vi "FisherPaykel Check GEA Inverter Selection.vi"(8 "Error In":errorcluster, 10 "Inverter ID":string(combo), 11 "Machine ID":string(combo)) -> (0 "Error Out":errorcluster, 3 "Throw Error?":bool)   [LabVIEW 2016]
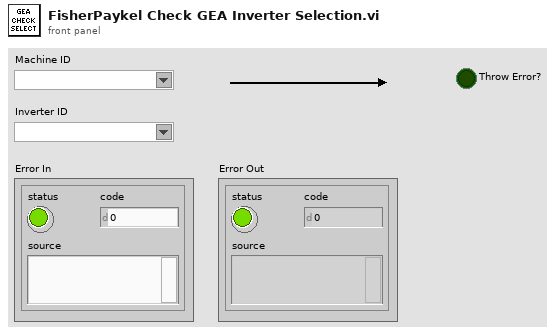
[diagram p1: front panel]
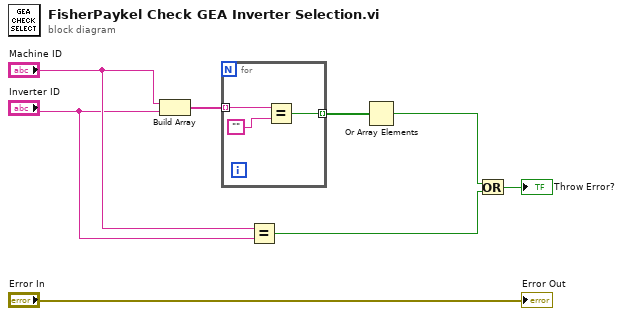
[diagram p0: block diagram]
diagram:
  n1 = Build Array("Machine ID", "Inverter ID") -> (w8:string[])
  n2 = for {
    tunnel: w8 -> [w11] mode=indexing
    tunnel: [w9] -> w5 mode=indexing
    n3 = Equal?(x=w11, y="") -> (x = y?=w9:bool)
  }
  n4 = Equal?(x="Machine ID", y="Inverter ID") -> (x = y?=w3:bool)
  n5 = Or Array Elements(Boolean array=w5) -> (logical OR=w4:bool)
  n6 = Or(x=w4, y=w3) -> (x .or. y?=→"Throw Error?":bool)
  "Error Out" <- "Error In"
